vi "DelayGeneratorGetState.vi"(9 "error in (no error)":errorcluster) -> (2 "State":T1, 6 "error out":errorcluster)   [LabVIEW 2009]
uses:
  Controls/DelayGeneratorState.ctl
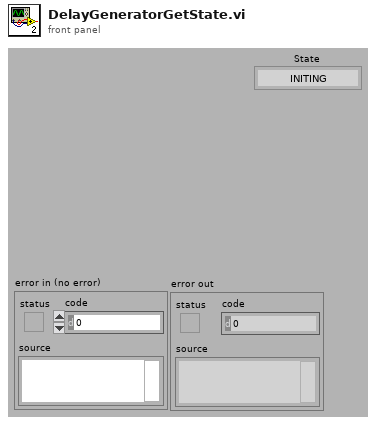
[diagram p1: front panel]
types:
  T1 = typedef "DelayGeneratorState.ctl" = enum16{"INITING", "IDLING", "TRACKING", "STOPPING"}
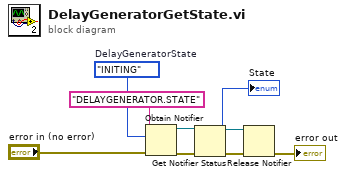
[diagram p0: block diagram]
diagram:
  w7 = DelayGeneratorState."INITING"  # DelayGeneratorState
  n1 = Obtain Notifier(name (unnamed)="DELAYGENERATOR.STATE", notification data type=w7, error in (no error)="error in (no error)") -> (notifier out=w5:refnum<notifier>, error out=w6:errorcluster)  [unwired: 1 in, 1 out]
  n2 = Get Notifier Status(notifier=w5, error in (no error)=w6) -> (notifier out=w3:refnum<notifier>, current notification=→"State":T1, error out=w4:errorcluster)  [unwired: 2 out]
  n3 = Release Notifier(notifier=w3, error in (no error)=w4) -> (error out=→"error out":errorcluster)  [unwired: 1 in, 2 out]
